vi "Execute.vi"(0 "reference in":refnum<class "SlideFeedCommand.lvclass">, 5 "error in (no error)":errorcluster) -> (14 "reference out":refnum<class "SlideFeedCommand.lvclass">, 19 "error out":errorcluster)   [LabVIEW 2013, in "SlideFeedCommand.lvclass"]
uses:
  SlideFeedCommand.lvclass
  Slide_class/Slide.lvclass
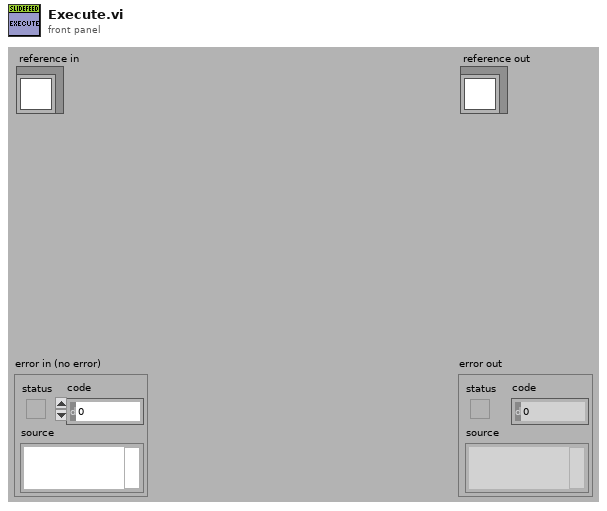
[diagram p1: front panel]
types:
  T1 = typedef "SlideFeedCommand.lvclass/ObjectAttributes.ctl" = cluster{"Slide.lvclass":refnum<class "Slide.lvclass">}
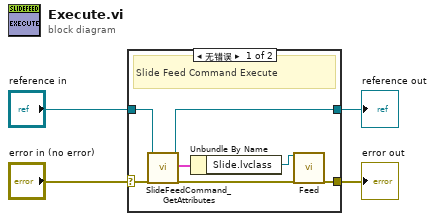
[diagram p0: block diagram]
diagram:
  n1 = case shown="无错误" "error in (no error)" {
    selector: "error in (no error)" -> [w11 w13]
    tunnel: [w5 w13] -> w3
    tunnel: [w10 w12] -> w1
    tunnel: "reference in" -> [w8 w12]
    frame No Error {
      # "Slide Feed Command Execute"
      n2 = call "SlideFeedCommand_GetAttributes.vi"("reference in"=w8, "error in (no error)"=w11) -> ("reference out"=w10:refnum<class "SlideFeedCommand.lvclass">, "attributes"=w9:T1, "error out"=w6:errorcluster)  [unwired: 14 in, 1 out]
      n3 = Unbundle By Name(w9) -> ("Slide.lvclass"=w7:refnum<class "Slide.lvclass">)
      n4 = call-dynamic "Feed.vi"("reference in"=w7, "error in (no error)"=w6) -> ("error out"=w5:errorcluster)  [unwired: 16 in, 1 out]
    }
    frame Error {
    }
  }
  "error out" <- w3
  "reference out" <- w1
